vi "Decimate Timeline graph data.vi"(9 "Data in":T1) -> (1 "Data out":T1)   [LabVIEW 2020]
uses:
  xcontrol/Interface VIs/Interface typedefs/Interface-Data format definition.ctl
  xcontrol/Typedefs/Xctl-XY data type definition.ctl
  xcontrol/Typedefs/Xctrl-ROI type enum.ctl
  xcontrol/Globals/gl_X-Grapher refs.vi
  xcontrol/XGrapher.xctl
panel:
  out "Output number of points":i32
  out "Nominal number of points shown in the graph":u32=2000
  out "# points in selected range":i32
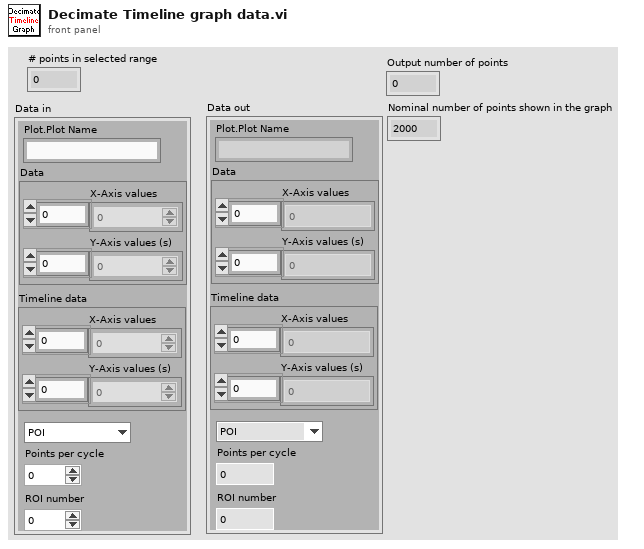
[diagram p1: front panel]
types:
  T1 = typedef "Interface-Data format definition.ctl" = cluster{"Plot.Plot Name":string, "Data":T2, "Timeline data":T2, "Type":T3, "Points per cycle":u16, "ROI number":u16}
  T2 = typedef "XGrapher.xctl/Xctl-XY data type definition.ctl" = cluster{"X-Axis values":sgl[], "Y-Axis values (s)":sgl[]}
  T3 = typedef "Xctrl-ROI type enum.ctl" = enum16{"POI", "Mini-scan", "Group"}
  T4 = typedef "XGrapher.xctl/Xctrl-Waveform graph ref.ctl" = refnum<vi>
  T5 = typedef "XGrapher.xctl/Xctrl-Timeline graph ref.ctl" = refnum<vi>
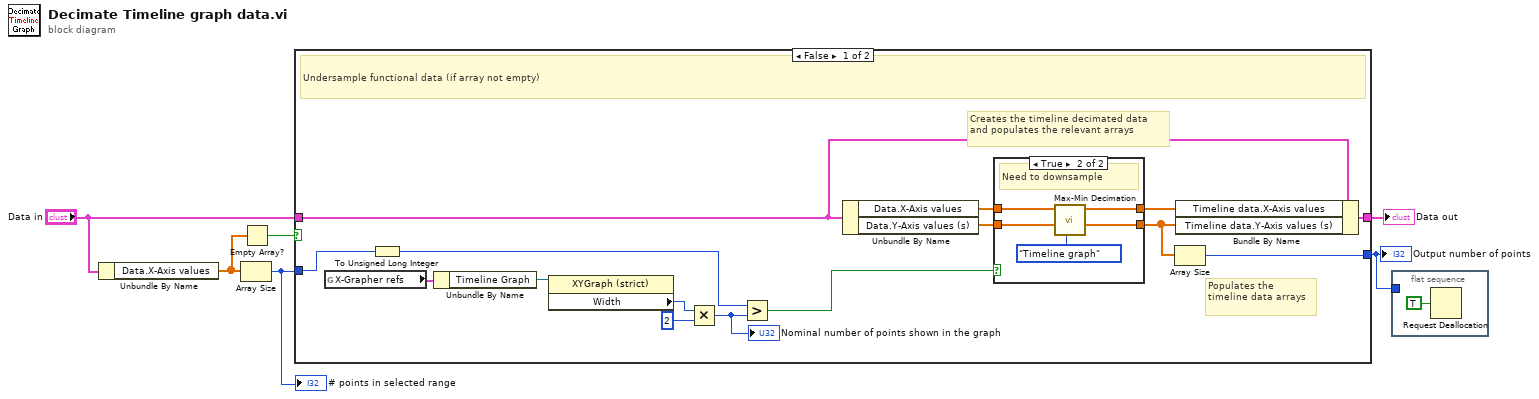
[diagram p0: block diagram]
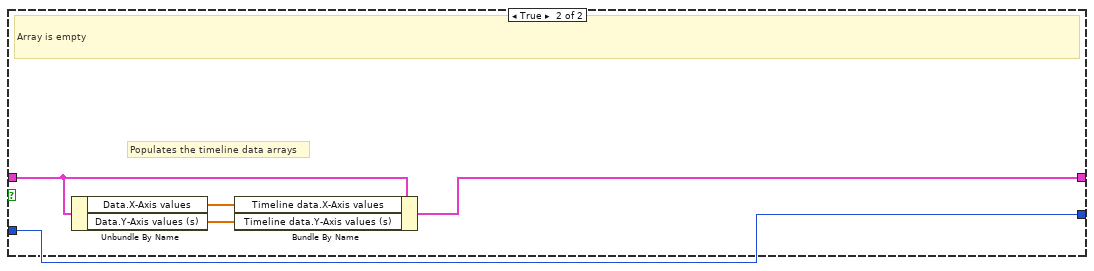
[diagram p3: hidden frame]
diagram:
  n1 = Unbundle By Name("Data in") -> ("Data.X-Axis values"=w3:sgl[])
  n2 = Array Size(array=w3) -> (size(s)=w2:i32)
  "# points in selected range" <- w2
  n3 = Empty Array?(array=w3) -> (empty?=w6:bool)
  n4 = case shown="False" w6 {
    tunnel: [w21 w30] -> w4
    tunnel: "Data in" -> [w11 w31]
    tunnel: [w8 w29] -> w1
    tunnel: w2 -> [w7 w29]
    frame False {
      # "Populates the timeline data arrays"
      # "Creates the timeline decimated data and populates the relevant arrays"
      # "Undersample functional data (if array not empty)"
      n5 = global read "gl_X-Grapher refs.vi" "X-Grapher refs"() -> (w17:cluster{"XY Graph":T4, "Timeline Graph":T5})
      n6 = To Unsigned Long Integer(number=w7) -> (unsigned 32bit integer=w10:u32)
      n7 = Unbundle By Name(w17) -> ("Timeline Graph"=w18:T5)
      n8 = property on="Property Node" class="XYGraph (strict)"(reference=w18) -> ("Width"=w20:u32)  [unwired: 1 in, 2 out]
      n9 = Multiply(x=w20, y=u32 2) -> (x*y=w16:u32)
      "Nominal number of points shown in the graph" <- w16
      n10 = Greater?(x=w10, y=w16) -> (0:w12:bool)
      n11 = Unbundle By Name(w11) -> ("Data.X-Axis values"=w15:sgl[], "Data.Y-Axis values (s)"=w14:sgl[])
      n12 = case shown="True" w12 {
        tunnel: w15 -> [w23 w28]
        tunnel: w14 -> [w22 w27]
        tunnel: [w23 w25] -> w13
        tunnel: [w22 w24] -> w9
        frame False {
        }
        frame True {
          # "Need to downsample"
          n13 = call "Max-Min Decimation.vi"("Which graph?"=enum16{"Main graph", "Timeline graph"}."Timeline graph", "Data.Y-Axis values"=w27, "Data.X-Axis values"=w28) -> ("Data.Y-Axis values"=w24:sgl[], "Data.X-Axis values"=w25:sgl[])  [unwired: 7 in]
        }
      }
      n14 = Array Size(array=w9) -> (size(s)=w8:i32)
      n15 = Bundle By Name(cluster=w11, "Timeline data.X-Axis values"=w13, "Timeline data.Y-Axis values (s)"=w9) -> (w21:T1)
    }
    frame True {
      # "Populates the timeline data arrays"
      # "Array is empty"
      n16 = Unbundle By Name(w31) -> ("Data.X-Axis values"=w33:sgl[], "Data.Y-Axis values (s)"=w32:sgl[])
      n17 = Bundle By Name(cluster=w31, "Timeline data.X-Axis values"=w33, "Timeline data.Y-Axis values (s)"=w32) -> (w30:T1)
    }
  }
  "Data out" <- w4
  "Output number of points" <- w1
  n18 = flat-sequence {
    tunnel: w1 -> [_]
    frame #0 {
      n19 = Request Deallocation(TRUE ("flag")) -> ()
    }
  }
